vi "Destroy.vi"(8 "error in (no error)":errorcluster, 11 "Current Value Table in":refnum<class "Current Value Table.lvclass">) -> (0 "error out":errorcluster)   [LabVIEW 2024, in "Current Value Table.lvlib" / "Current Value Table.lvclass"]
uses:
  Current Value Table.lvclass
  Current Value Table.lvclass/Current Value Table.ctl
  iCVT_Item/iCVT_Item.lvclass
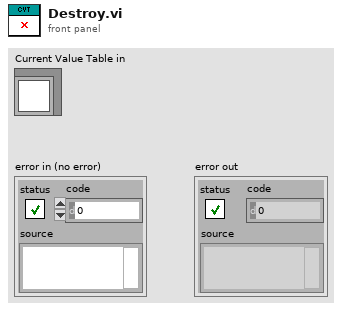
[diagram p1: front panel]
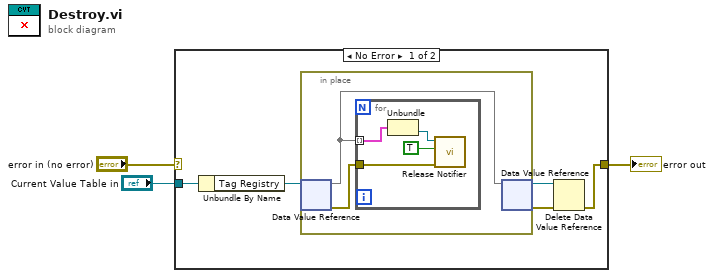
[diagram p0: block diagram]
diagram:
  n1 = case shown="No Error" "error in (no error)" {
    selector: "error in (no error)" -> [_ w15]
    tunnel: [w4 w15] -> w2
    tunnel: "Current Value Table in" -> [w8 _]
    frame No Error {
      n2 = Unbundle By Name(w8) -> ("Tag Registry"=w7:refnum<data-value>)
      n3 = in-place {
        n4 = in-place-dvr #1(w7) -> (w10:map{string, refnum<class "iCVT_Item.lvclass">}, w9:errorcluster)
        n5 = for {
          tunnel: w10 -> [w14] mode=indexing
          tunnel: w9 -> [w11]
          n6 = Unbundle(w14) -> ("Current Value Table.lvlib:iCVT_Item.lvclass"=w13:refnum<class "iCVT_Item.lvclass">)  [unwired: 1 out]
          n7 = call-dynamic "Release Notifier.vi"("error in (no error)"=w11, "force destroy? (F)"=TRUE, "iCVT_Item in"=w13) -> ()  [unwired: 7 in, 2 out]
        }
        n8 = in-place-dvr #1(w10) -> (w6:refnum<data-value>, w5:errorcluster)
      }
      n9 = Delete Data Value Reference(data value reference=w6, error in=w5) -> (error out=w4:errorcluster)  [unwired: 1 out]
    }
    frame Error {
    }
  }
  "error out" <- w2
